vi "Test Coffee Shop List Baristas.vi"(8 "error in (no error)":errorcluster, 11 "Coffee Shop Test In":refnum<class "Coffee Shop Test.lvclass">=refnum) -> (0 "error out":errorcluster, 3 "Coffee Shop Test Out":refnum<class "Coffee Shop Test.lvclass">)   [LabVIEW 2020, in "Coffee Shop Test.lvclass"]
uses:
  Coffee Shop Test.lvclass
  Processes/Coffee Shop/Coffee Shop.lvclass
  <vilib>/Astemes/Triarc Framework/Process/Process.lvclass
  C:/Program Files (x86)/National Instruments/LabVIEW 2020/vi.lib/Astemes/Triarc Framework/Application/Application.lvclass
  C:/Program Files (x86)/National Instruments/LabVIEW 2020/vi.lib/Astemes/Triarc Framework/Process/Process.lvclass
  C:/Program Files (x86)/National Instruments/LabVIEW 2020/vi.lib/Astemes/Triarc Framework/Base/Base.lvclass
  C:/Program Files (x86)/National Instruments/LabVIEW 2020/vi.lib/Astemes/Triarc Framework/Error Handler Interface/Error Handler Interface.lvclass
  C:/Program Files (x86)/National Instruments/LabVIEW 2020/vi.lib/Astemes/Triarc Framework/Logging/Logging.lvclass
  C:/Program Files (x86)/National Instruments/LabVIEW 2020/vi.lib/Astemes/Triarc Framework/Async Handler/Async Handler.lvclass
  C:/git/astemes-triarc-examples/source/Coffee Shop/Processes/Coffee Shop/Coffee Shop.lvclass
  5ca4e339-37d4-4178-8edf-2602ad112828.vi
  <vilib>/Astemes/LUnit/Test Case.lvclass
  C:/Program Files (x86)/National Instruments/LabVIEW 2020/vi.lib/Astemes/LUnit/Test Case.lvclass
  C:/Program Files (x86)/National Instruments/LabVIEW 2020/vi.lib/Astemes/LUnit/LUnit Runnable.lvclass
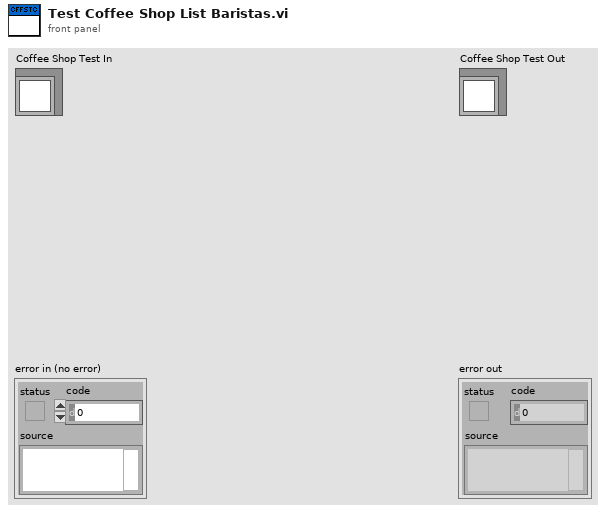
[diagram p1: front panel]
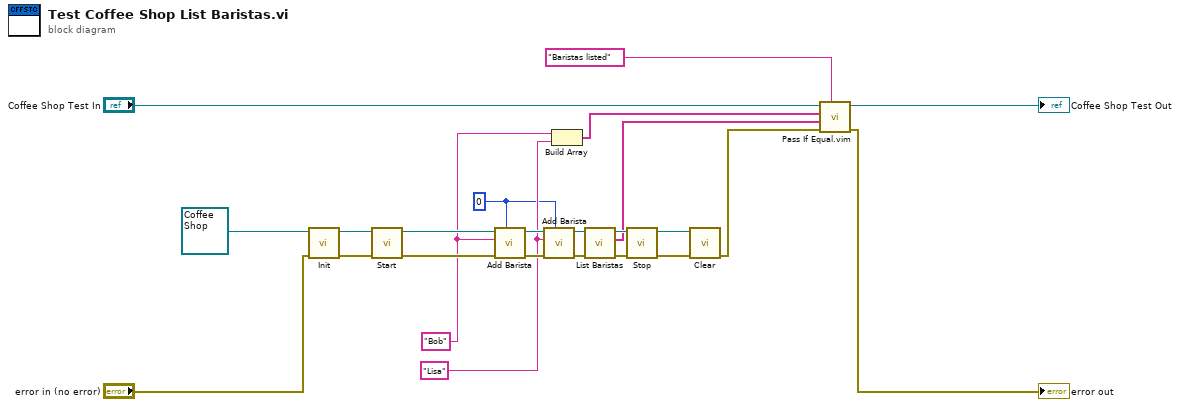
[diagram p0: block diagram]
diagram:
  w1 = u32 0 ("Time Scale [ms]")
  w4 = "Lisa"
  w5 = "Bob" ("Name")
  n1 = call-dynamic "Init.vi"("error in (no error)"="error in (no error)", "Process In"=refnum<class "Coffee Shop.lvclass"> refnum ("Coffee Shop.lvclass")) -> ("error out"=w22:errorcluster, "Process Out"=w23:refnum<class "Coffee Shop.lvclass">)  [unwired: 8 in]
  n2 = call <vilib>:"Start.vi"("error in (no error)"=w22, "Process In"=w23) -> ("error out"=w17:errorcluster, "Process Out"=w16:refnum<class "Coffee Shop.lvclass">)  [unwired: 7 in, 1 out]
  n3 = call "Add Barista.vi"("Time Scale [ms]"=w1, "error in (no error)"=w17, "Name"=w5, "Coffee Shop in"=w16) -> ("error out"=w18:errorcluster, "Coffee Shop out"=w9:refnum<class "Coffee Shop.lvclass">)  [unwired: 6 in]
  n4 = call "Add Barista.vi"("Time Scale [ms]"=w1, "error in (no error)"=w18, "Name"=w4, "Coffee Shop in"=w9) -> ("error out"=w10:errorcluster, "Coffee Shop out"=w7:refnum<class "Coffee Shop.lvclass">)  [unwired: 6 in]
  n5 = Build Array(w5, w4) -> (w3:string[])
  n6 = call "List Baristas.vi"("error in (no error)"=w10, "Coffee Shop in"=w7) -> ("error out"=w8:errorcluster, "Names"=w2:string[], "Coffee Shop out"=w6:refnum<class "Coffee Shop.lvclass">)  [unwired: 7 in]
  n7 = call <vilib>:"Stop.vi"("error in (no error)"=w8, "Process In"=w6) -> ("error out"=w20:errorcluster, "Process Out"=w21:refnum<class "Coffee Shop.lvclass">)  [unwired: 7 in, 1 out]
  n8 = call-dynamic "Clear.vi"("error in (no error)"=w20, "Application In"=w21) -> ("error out"=w13:errorcluster)  [unwired: 9 in]
  n9 = call "Pass If Equal.vim"("Description"="Baristas listed", "error in (no error)"=w13, "Actual"=w2, "Expected"=w3, "LUnit Test Case In"="Coffee Shop Test In") -> ("error out"=→"error out":errorcluster, "LUnit Test Case Out"=→"Coffee Shop Test Out":refnum<class "Test Case.lvclass">)  [unwired: 5 in]
